vi "TdmsIcons_OpenFile.vi"(8 "error in (no error)":errorcluster, 11 "Path":path) -> (0 "error out":errorcluster, 3 "TdmsOut":refnum<k34>)   [LabVIEW 2014]
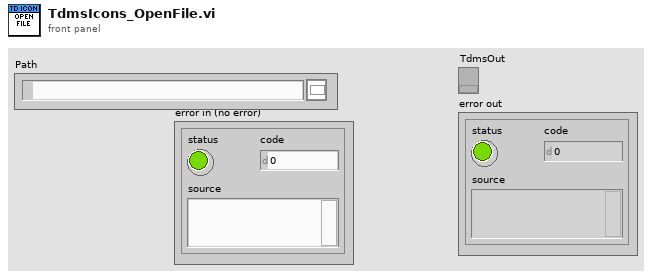
[diagram p1: front panel]
types:
  T1 = enum16{"open", "open or create", "create or replace", "create", "open (read-only)"}
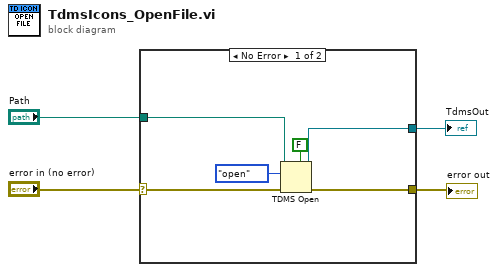
[diagram p0: block diagram]
diagram:
  n1 = case shown="No Error" "error in (no error)" {
    selector: "error in (no error)" -> [w8 w11]
    tunnel: [w5 _] -> w4
    tunnel: [w7 w11] -> w3
    tunnel: "Path" -> [w6 _]
    frame No Error {
      n2 = TDMS Open(5:FALSE ("create index file? (T)"), 8:w8, 10:T1."open" ("operation (0:open)"), 11:w6) -> (0:w7:errorcluster, 3:w5:refnum<k34>)  [unwired: 3 in]
    }
    frame Error {
    }
  }
  "TdmsOut" <- w4
  "error out" <- w3
